vi "loadDataNodeBegin.vi"(8 "error in (no error)":errorcluster, 10 "XML Refnum in":refnum<file>, 11 "Category in":refnum<class "Category.lvclass">) -> (0 "error out":errorcluster, 2 "XML Refnum out":refnum<file>, 3 "Category out":refnum<class "Category.lvclass">)   [LabVIEW 2013, in "Category.lvclass"]
doc: "Part of the file loading process. Occurs at the beginning of a node being loaded. Loads the common xceDataNode data name and description."
uses:
  Category.lvclass
  xCE/xceDataNode/xceDataNode.lvclass
  XML Parser/XML Parser.lvclass
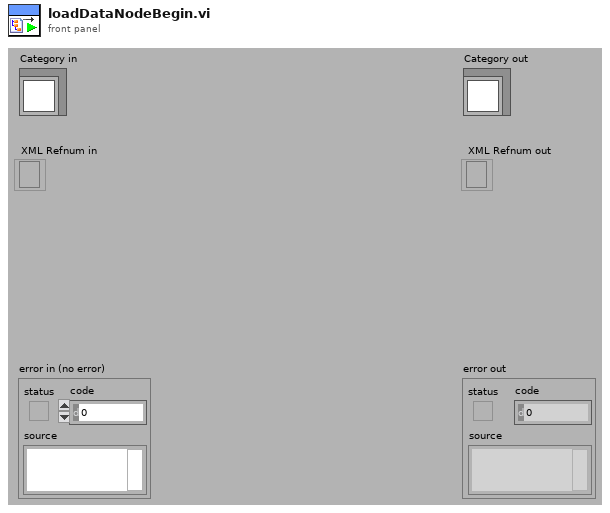
[diagram p1: front panel]
types:
  T1 = typedef "enum_Symbols.ctl" = enum16{"Default", "Analog Input", "Analog Output", "Digital Input", "Digital Output", "PWM Input", "PWM Output"}
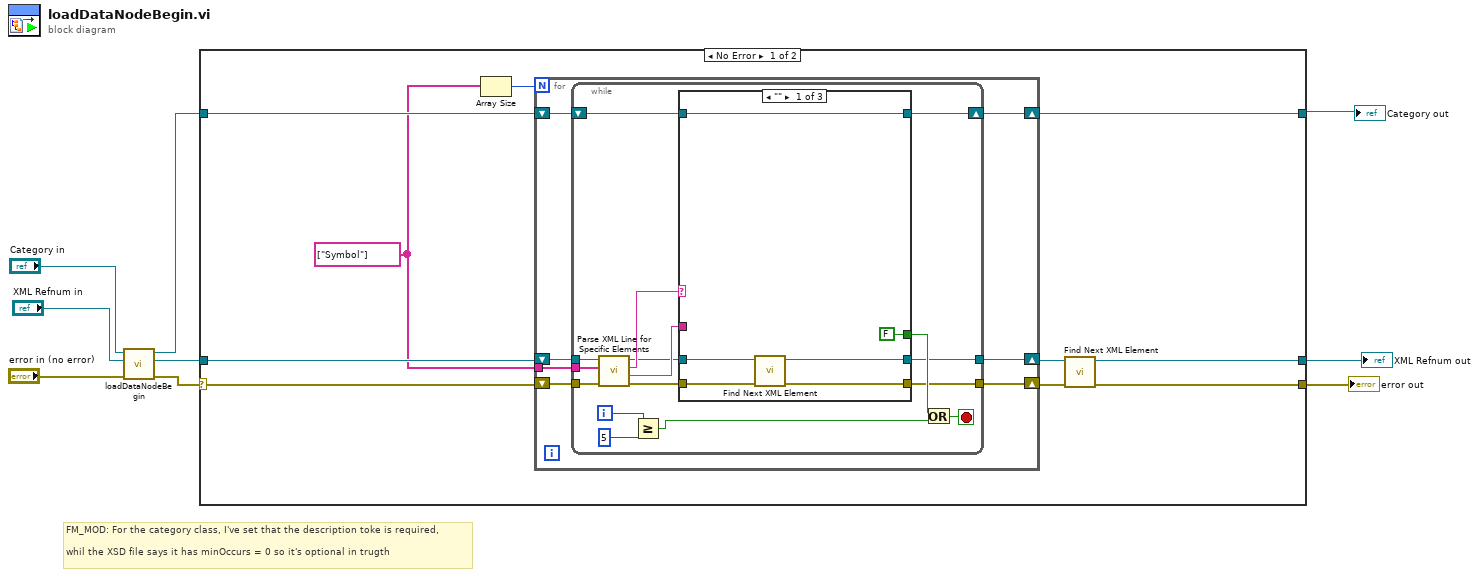
[diagram p0: block diagram]
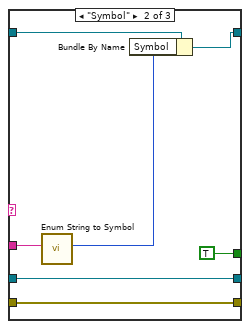
[diagram p2: hidden frame]
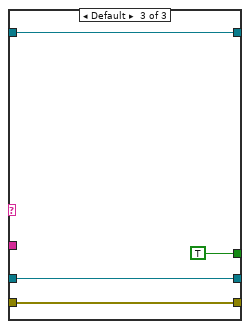
[diagram p3: hidden frame]
diagram:
  # "FM_MOD: For the category class, I've set that the description toke is required,\n\nwhil the XSD file says it has minOccurs = 0 so it's optional in trugth"
  n1 = call-parent "loadDataNodeBegin.vi"("error in (no error)"="error in (no error)", "XML Refnum in"="XML Refnum in", "xceDataNode in"="Category in") -> ("error out"=w6:errorcluster, "XML Refnum out"=w4:refnum<file>, "xceDataNode out"=w5:refnum<class "Category.lvclass">)  [unwired: 6 in]
  n2 = case shown="No Error" w6 {
    selector: w6 -> [w16 w61]
    tunnel: w5 -> [w18 w62]
    tunnel: w4 -> [w17 w60]
    tunnel: [w11 w60] -> w3
    tunnel: [w10 w61] -> w2
    tunnel: [w15 w62] -> w1
    frame No Error {
      w12 = string[] ["Symbol"]
      n3 = Array Size(array=w12) -> (size(s)=w19:i32)
      n4 = for {
        N: w19 -> [_]
        tunnel: w12 -> [w26]
        shift-right: [w21] -> w15
        shift-left: w18 -> [w23]
        shift-right: [w22] -> w14
        shift-left: w17 -> [w25]
        shift-right: [w20] -> w13
        shift-left: w16 -> [w24]
        n5 = while {
          tunnel: w26 -> [w42]
          tunnel: w25 -> [w41]
          tunnel: w24 -> [w40]
          shift-right: [w35] -> w21
          shift-left: w23 -> [w37]
          tunnel: [w27] -> w22
          tunnel: [w28] -> w20
          i -> [w39]
          stop <- w32 stop-if-true
          n6 = call "Parse XML Line for Specific Elements.vi"("error in (no error)"=w40, "Elements"=w42, "XML Refnum in"=w41) -> ("error out"=w29:errorcluster, "Value"=w31:string, "Element Name"=w36:string, "XML Refnum out"=w30:refnum<file>)  [unwired: 4 in, 1 out]
          n7 = Greater Or Equal?(x=w39, y=5) -> (x >= y?=w33:bool)
          n8 = case shown="\"\"" w36 {
            tunnel: w37 -> [w48 w55 w59]
            tunnel: [w48 w54 w59] -> w35
            tunnel: [FALSE TRUE TRUE] -> w34
            tunnel: w31 -> [_ w50 _]
            tunnel: w30 -> [w46 w52 w57]
            tunnel: w29 -> [w44 w51 w56]
            tunnel: [w43 w51 w56] -> w28
            tunnel: [w45 w52 w57] -> w27
            frame "" {
              n9 = call "Find Next XML Element.vi"("error in (no error)"=w44, "XML Fine In"=w46) -> ("error out"=w43:errorcluster, "XML Fine Out"=w45:refnum<file>)  [unwired: 7 in, 1 out]
            }
            frame "Symbol" {
              n10 = call "Enum String to Symbol.vi"("Symbol String In"=w50) -> ("Symbol Enum Out"=w49:T1)  [unwired: 10 in]
              n11 = Bundle By Name(cluster=w55, "Symbol"=w49) -> (w54:refnum<class "Category.lvclass">)
            }
            frame Default {
            }
          }
          n12 = Or(x=w34, y=w33) -> (x .or. y?=w32:bool)
        }
      }
      n13 = call "Find Next XML Element.vi"("error in (no error)"=w13, "XML Fine In"=w14) -> ("error out"=w10:errorcluster, "XML Fine Out"=w11:refnum<file>)  [unwired: 7 in, 1 out]
    }
    frame Error {
    }
  }
  "error out" <- w2
  "Category out" <- w1
  "XML Refnum out" <- w3
